vi "Extract Tip Features.vi"() -> ()   [LabVIEW 2013]
uses:
  <vilib>/Utility/file.llb/Write To Spreadsheet File (DBL).vi
panel:
  in  "Non-tip Data File":path=path "C:/Users/Andrew/Documents/Apatite to Zircon Code/Track Finding/Non-tip Data.csv"
  in  "Tip Data File":path=path "C:/Users/Andrew/Documents/Apatite to Zircon Code/Track Finding/Tip Data.csv"
  out "error out":errorcluster
  in  "error in (no error)":errorcluster
  in  "Non-tips Root":path=path "C:/Users/Andrew/Documents/Apatite to Zircon Code/Track Finding/Tip Images/Non-Tips"
  in  "Tips Root":path=path "C:/Users/Andrew/Documents/Apatite to Zircon Code/Track Finding/Tip Images/Tips"
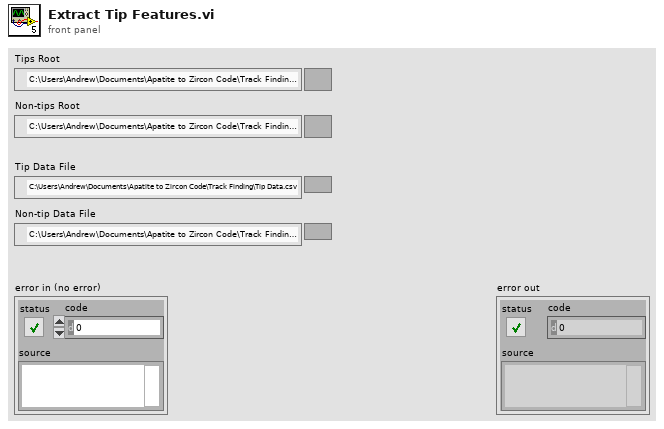
[diagram p1: front panel]
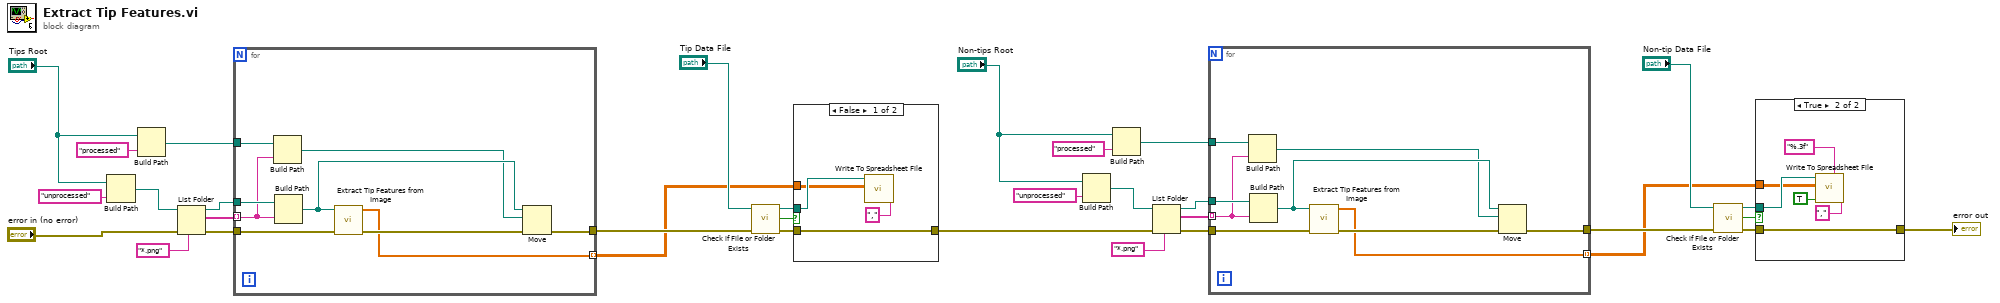
[diagram p0: block diagram]
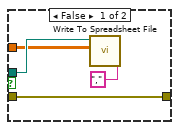
[diagram p2: hidden frame]
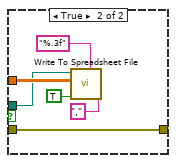
[diagram p3: hidden frame]
diagram:
  n1 = Build Path(base path="Tips Root", name or relative path="unprocessed") -> (appended path=w26:path)
  n2 = Build Path(base path="Tips Root", name or relative path="processed") -> (appended path=w21:path)
  n3 = List Folder(path=w26, pattern="*.png", error in="error in (no error)") -> (path out=w24:path, filenames=w25:string[], error out=w31:errorcluster)  [unwired: 1 in, 1 out]
  n4 = for {
    tunnel: w31 -> [w42]
    tunnel: w25 -> [w38] mode=indexing
    tunnel: w24 -> [w41]
    tunnel: w21 -> [w39]
    tunnel: [w35] -> w11 mode=indexing
    tunnel: [w34] -> w13
    n5 = Build Path(base path=w39, name or relative path=w38) -> (appended path=w37:path)
    n6 = Build Path(base path=w41, name or relative path=w38) -> (appended path=w40:path)
    n7 = call "Extract Tip Features from Image.vi"("error in (no error)"=w42, "Image Path"=w40) -> ("error out"=w36:errorcluster, "Features"=w35:dbl[])  [unwired: 8 in]
    n8 = Move(source path=w40, error in=w36, 10:w37) -> (error out=w34:errorcluster)  [unwired: 2 in, 2 out]
  }
  n9 = call <vilib>:"Check if File or Folder Exists.vi"("error in (no error)"=w13, "path"="Tip Data File") -> ("error out"=w28:errorcluster, "file or folder exists?"=w29:bool, "dup path"=w30:path)  [unwired: 7 in]
  n10 = case shown="False" w29 {
    tunnel: w11 -> [w44 w50]
    tunnel: w28 -> [w45 w48]
    tunnel: w30 -> [w46 w49]
    tunnel: [w45 w48] -> w10
    frame False {
      n11 = call-poly <vilib>:"Write To Spreadsheet File.vi"("delimiter (\\t)"="," ("delimiter (\\t)"), "2D data"=w44, "file path (dialog if empty)"=w46) -> ()  [unwired: 5 in, 1 out]
    }
    frame True {
      n12 = call-poly <vilib>:"Write To Spreadsheet File.vi"("delimiter (\\t)"="," ("delimiter (\\t)"), "format (%.3f)"="%.3f", "append to file? (new file:F)"=TRUE, "2D data"=w50, "file path (dialog if empty)"=w49) -> ()  [unwired: 3 in, 1 out]
    }
  }
  n13 = Build Path(base path="Non-tips Root", name or relative path="unprocessed") -> (appended path=w18:path)
  n14 = Build Path(base path="Non-tips Root", name or relative path="processed") -> (appended path=w14:path)
  n15 = List Folder(path=w18, pattern="*.png", error in=w10) -> (path out=w16:path, filenames=w17:string[], error out=w19:errorcluster)  [unwired: 1 in, 1 out]
  n16 = for {
    tunnel: w19 -> [w61]
    tunnel: w17 -> [w57] mode=indexing
    tunnel: w16 -> [w60]
    tunnel: w14 -> [w58]
    tunnel: [w54] -> w3 mode=indexing
    tunnel: [w53] -> w4
    n17 = Build Path(base path=w58, name or relative path=w57) -> (appended path=w56:path)
    n18 = Build Path(base path=w60, name or relative path=w57) -> (appended path=w59:path)
    n19 = call "Extract Tip Features from Image.vi"("error in (no error)"=w61, "Image Path"=w59) -> ("error out"=w55:errorcluster, "Features"=w54:dbl[])  [unwired: 8 in]
    n20 = Move(source path=w59, error in=w55, 10:w56) -> (error out=w53:errorcluster)  [unwired: 2 in, 2 out]
  }
  n21 = call <vilib>:"Check if File or Folder Exists.vi"("error in (no error)"=w4, "path"="Non-tip Data File") -> ("error out"=w7:errorcluster, "file or folder exists?"=w8:bool, "dup path"=w9:path)  [unwired: 7 in]
  n22 = case shown="True" w8 {
    tunnel: w7 -> [w64 w68]
    tunnel: w9 -> [w65 w69]
    tunnel: [w64 w68] -> w5
    tunnel: w3 -> [w62 w66]
    frame False {
      n23 = call-poly <vilib>:"Write To Spreadsheet File.vi"("delimiter (\\t)"="," ("delimiter (\\t)"), "2D data"=w62, "file path (dialog if empty)"=w65) -> ()  [unwired: 5 in, 1 out]
    }
    frame True {
      n24 = call-poly <vilib>:"Write To Spreadsheet File.vi"("delimiter (\\t)"="," ("delimiter (\\t)"), "format (%.3f)"="%.3f", "append to file? (new file:F)"=TRUE, "2D data"=w66, "file path (dialog if empty)"=w69) -> ()  [unwired: 3 in, 1 out]
    }
  }
  "error out" <- w5
